vi "ValidateConfig.vi"(8 "error in (no error)":errorcluster, 11 "Channel in":refnum<class "Channel.lvclass">) -> (0 "error out":errorcluster, 2 "valid?":bool, 3 "Channel out":refnum<class "Channel.lvclass">)   [LabVIEW 2018, in "Channel.lvclass"]
uses:
  Channel.lvclass
  Channel.lvclass/Channel.ctl
  Interface/Interface.lvclass/Interface.ctl
  Interface/Interface.lvclass
panel:
  # "T=valid\nF=error"
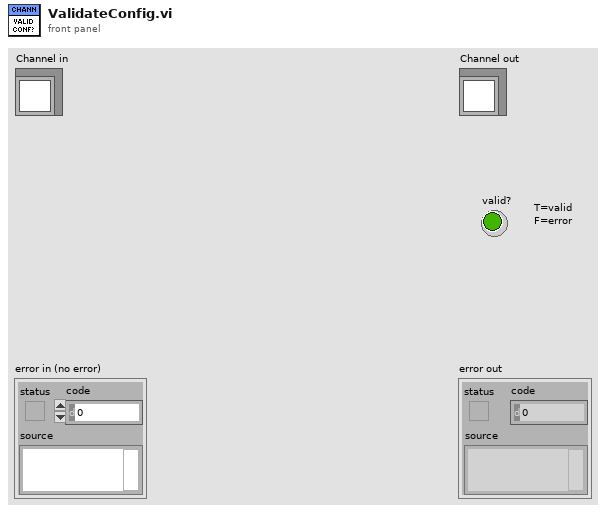
[diagram p1: front panel]
types:
  T1 = cluster{"ACQUISITION_MODE":u8, "TRIGGER_MODE":u8, "READ_MODE":u8, "PREAMP":u8, "READOUT_RATE":u8, "VERTICAL_SHIFT_SPEED":u8, "EM_MODE":u8, "EM_GAIN":u16, "SHUTTER_MODE":u8, "SHUTTER_TTL":u8, "SHUTTER_OPENING_TIME":u16, "SHUTTER_CLOSING_TIME":u16, "VBIN":u16, "HBIN":u16, "INITIAL_LINE":u16, "INITIAL_COLUMN":u16, "FINAL_LINE":u16, "FINAL_COLUMN":u16, "FRAME_TRANSFER":bool, "VERTICAL_CLOCK_VOLTAGE":u8, "AD_CHANNEL":u32}
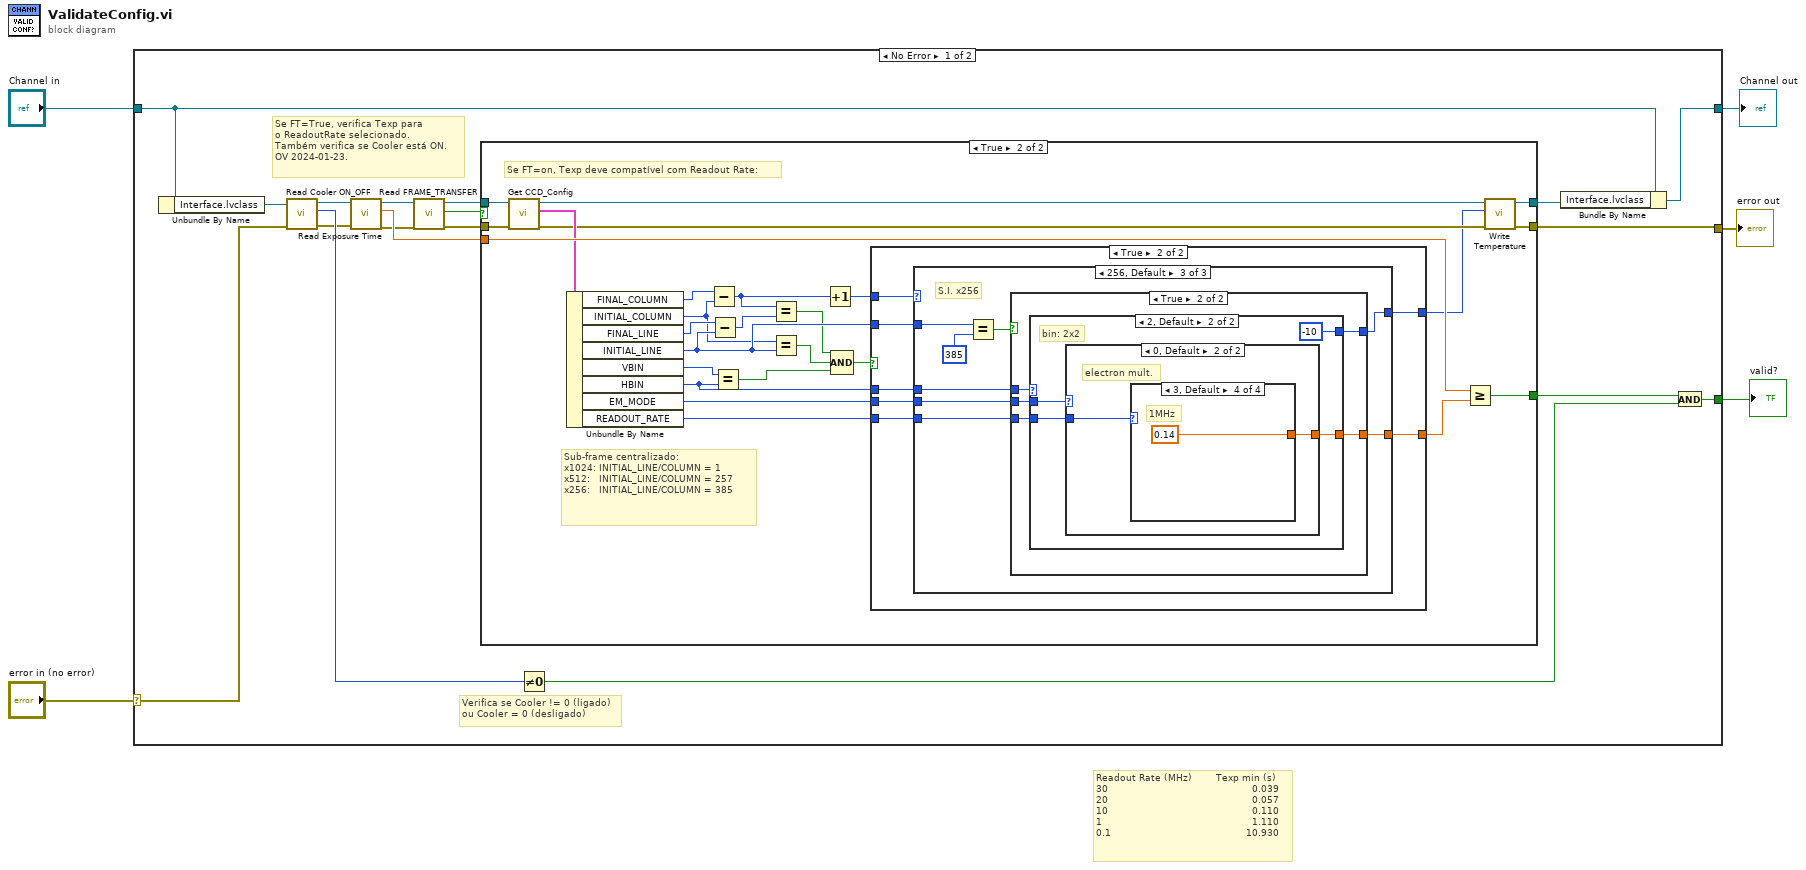
[diagram p0: block diagram]
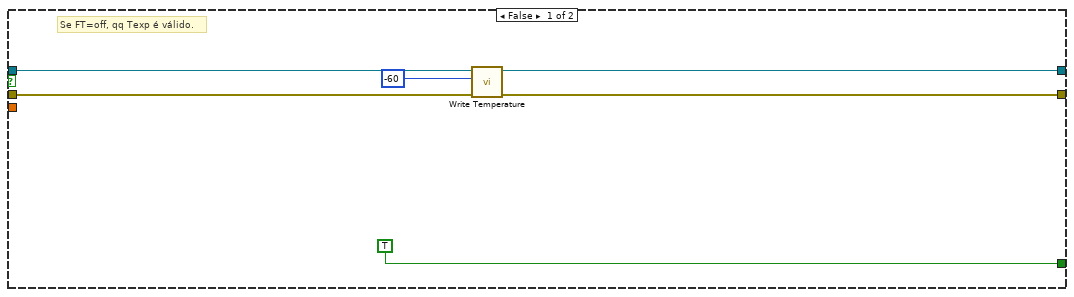
[diagram p2: hidden frame]
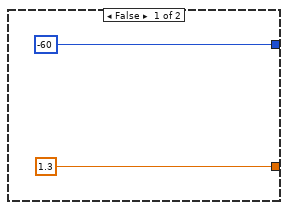
[diagram p3: hidden frame]
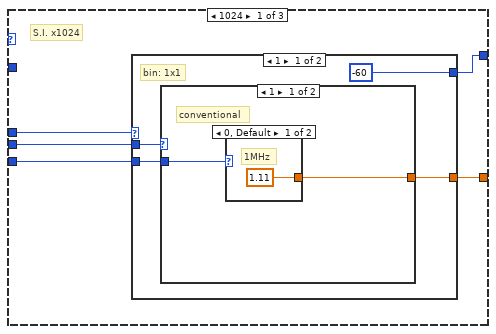
[diagram p4: hidden frame]
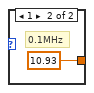
[diagram p5: hidden frame]
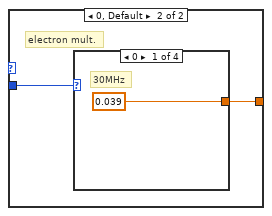
[diagram p6: hidden frame]
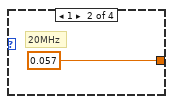
[diagram p7: hidden frame]
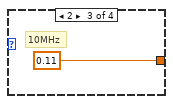
[diagram p8: hidden frame]
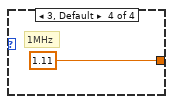
[diagram p9: hidden frame]
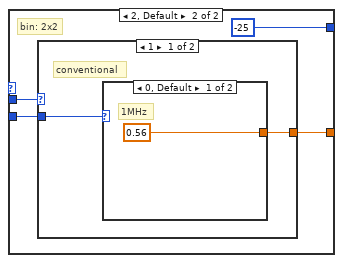
[diagram p10: hidden frame]
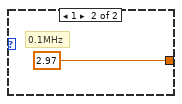
[diagram p11: hidden frame]
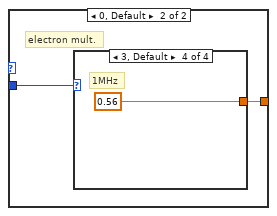
[diagram p12: hidden frame]
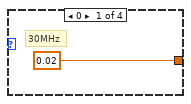
[diagram p13: hidden frame]
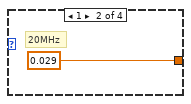
[diagram p14: hidden frame]
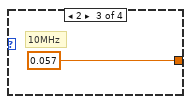
[diagram p15: hidden frame]
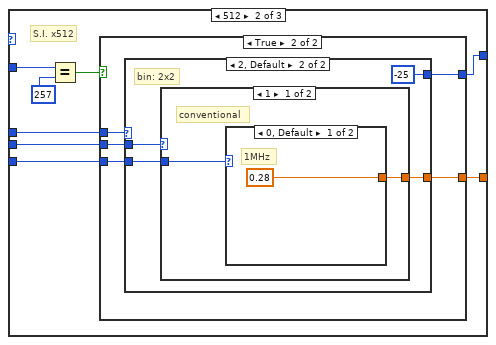
[diagram p16: hidden frame]
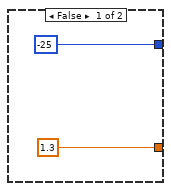
[diagram p17: hidden frame]
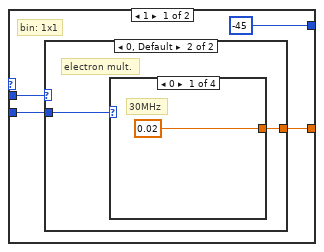
[diagram p18: hidden frame]
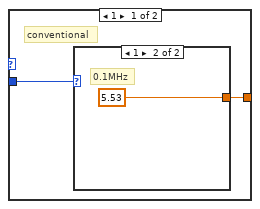
[diagram p19: hidden frame]
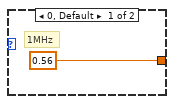
[diagram p20: hidden frame]
diagram:
  # "Readout Rate (MHz)        Texp min (s)\n30                                                0.039\n20                                                0.057  \n10                                                0.110\n1                                                  1.110\n0.1                                             10.930"
  n1 = case shown="No Error" "error in (no error)" {
    selector: "error in (no error)" -> [w17 w186]
    tunnel: [w9 w186] -> w4
    tunnel: [w7 w185] -> w2
    tunnel: "Channel in" -> [w8 w185]
    tunnel: [w14 FALSE] -> w1
    frame No Error {
      # "Verifica se Cooler != 0 (ligado)\nou Cooler = 0 (desligado)"
      # "Se FT=True, verifica Texp para \no ReadoutRate selecionado.\nTambém verifica se Cooler está ON.\nOV 2024-01-23."
      n2 = Unbundle By Name(w8) -> ("Interface.lvclass"=w20:refnum<class "Interface.lvclass">)
      n3 = call-dynamic "Read Cooler ON_OFF.vi"("error in (no error)"=w17, "Interface in"=w20) -> ("error out"=w16:errorcluster, "Cooler ON/OFF"=w18:i16, "Interface out"=w19:refnum<class "Interface.lvclass">)  [unwired: 7 in]
      n4 = call "Read Exposure Time.vi"("error in (no error)"=w16, "Interface in"=w19) -> ("error out"=w15:errorcluster, "Exposure Time"=w21:dbl, "Interface out"=w23:refnum<class "Interface.lvclass">)  [unwired: 7 in]
      n5 = call-dynamic "Read FRAME_TRANSFER.vi"("error in (no error)"=w15, "Interface in"=w23) -> ("error out"=w10:errorcluster, "FRAME_TRANSFER"=w22:bool, "Interface out"=w11:refnum<class "Interface.lvclass">)  [unwired: 7 in]
      n6 = case shown="True" w22 {
        tunnel: w21 -> [_ w55]
        tunnel: [TRUE w53] -> w13
        tunnel: w11 -> [w27 w51]
        tunnel: w10 -> [w28 w50]
        tunnel: [w25 w37] -> w9
        tunnel: [w26 w34] -> w6
        frame False {
          # "Se FT=off, qq Texp é válido."
          n7 = call-dynamic "Write Temperature.vi"("error in (no error)"=w28, "Temperature"=i8 -60, "Interface in"=w27) -> ("error out"=w25:errorcluster, "Interface out"=w26:refnum<class "Interface.lvclass">)  [unwired: 7 in]
        }
        frame True {
          # "Sub-frame centralizado:\nx1024: INITIAL_LINE/COLUMN = 1\nx512:   INITIAL_LINE/COLUMN = 257\nx256:   INITIAL_LINE/COLUMN = 385"
          # "Se FT=on, Texp deve compatível com Readout Rate:"
          n8 = call-dynamic "Get CCD_Config.vi"("error in (no error)"=w50, "Interface in"=w51) -> ("error out"=w38:errorcluster, "output cluster"=w52:T1, "Interface out"=w35:refnum<class "Interface.lvclass">)  [unwired: 7 in]
          n9 = Unbundle By Name(w52) -> ("FINAL_COLUMN"=w47:u16, "INITIAL_COLUMN"=w32:u16, "FINAL_LINE"=w46:u16, "INITIAL_LINE"=w33:u16, "VBIN"=w44:u16, "HBIN"=w40:u16, "EM_MODE"=w49:u8, "READOUT_RATE"=w48:u8)
          n10 = Subtract(x=w47, y=w32) -> (x-y=w41:u16)
          n11 = Subtract(x=w46, y=w33) -> (x-y=w45:u16)
          n12 = Equal?(x=w44, y=w40) -> (x = y?=w42:bool)
          n13 = Equal?(x=w41, y=w45) -> (x = y?=w31:bool)
          n14 = Equal?(x=w32, y=w33) -> (x = y?=w30:bool)
          n15 = Increment(x=w41) -> (x+1=w39:u16)
          n16 = Compound Arithmetic op=AND(w31, w30, w42) -> (w43:bool)
          n17 = case shown="True" w43 {
            tunnel: [1.3 ("y") w64] -> w54
            tunnel: w49 -> [_ w63]
            tunnel: w48 -> [_ w62]
            tunnel: w39 -> [_ w61]
            tunnel: w40 -> [_ w60]
            tunnel: [i8 -60 ("y") w59] -> w36
            tunnel: w33 -> [_ w58]
            frame False {
            }
            frame True {
              n18 = case shown="256, Default" w61 {
                tunnel: [w69 w105 w148] -> w64
                tunnel: w63 -> [w68 w104 w147]
                tunnel: w62 -> [w67 w103 w146]
                tunnel: w60 -> [w66 w102 w145]
                tunnel: [w65 w101 w144] -> w59
                tunnel: w58 -> [_ w100 w142]
                frame 1024 {
                  # "S.I. x1024"
                  n19 = case shown="1" w66 {
                    tunnel: [w73 w87] -> w69
                    tunnel: w68 -> [w72 w86]
                    tunnel: w67 -> [w71 w85]
                    tunnel: [i8 -60 ("y") i8 -25 ("y")] -> w65
                    frame 1 {
                      # "bin: 1x1"
                      n20 = case shown="1" w72 {
                        tunnel: [w75 w79] -> w73
                        tunnel: w71 -> [w74 w78]
                        frame 1 {
                          # "conventional"
                          n21 = case shown="0, Default" w74 {
                            tunnel: [1.11 ("y") 10.93 ("y")] -> w75
                            frame 0, Default {
                              # "1MHz"
                            }
                            frame 1 {
                              # "0.1MHz"
                            }
                          }
                        }
                        frame 0, Default {
                          # "electron mult."
                          n22 = case shown="0" w78 {
                            tunnel: [0.039 ("y") 0.057 ("y") 0.11 ("y") 1.11 ("y")] -> w79
                            frame 0 {
                              # "30MHz"
                            }
                            frame 1 {
                              # "20MHz"
                            }
                            frame 2 {
                              # "10MHz"
                            }
                            frame 3, Default {
                              # "1MHz"
                            }
                          }
                        }
                      }
                    }
                    frame 2, Default {
                      # "bin: 2x2"
                      n23 = case shown="1" w86 {
                        tunnel: [w89 w93] -> w87
                        tunnel: w85 -> [w88 w92]
                        frame 1 {
                          # "conventional"
                          n24 = case shown="0, Default" w88 {
                            tunnel: [0.56 ("y") 2.97 ("y")] -> w89
                            frame 0, Default {
                              # "1MHz"
                            }
                            frame 1 {
                              # "0.1MHz"
                            }
                          }
                        }
                        frame 0, Default {
                          # "electron mult."
                          n25 = case shown="3, Default" w92 {
                            tunnel: [0.02 ("y") 0.029 ("y") 0.057 ("y") 0.56 ("y")] -> w93
                            frame 0 {
                              # "30MHz"
                            }
                            frame 1 {
                              # "20MHz"
                            }
                            frame 2 {
                              # "10MHz"
                            }
                            frame 3, Default {
                              # "1MHz"
                            }
                          }
                        }
                      }
                    }
                  }
                }
                frame 512 {
                  # "S.I. x512"
                  n26 = Equal?(x=w100, y=u16 257) -> (x = y?=w98:bool)
                  n27 = case shown="True" w98 {
                    tunnel: [1.3 ("y") w112] -> w105
                    tunnel: w104 -> [_ w111]
                    tunnel: w103 -> [_ w110]
                    tunnel: w102 -> [_ w109]
                    tunnel: [i8 -25 ("y") w108] -> w101
                    frame False {
                    }
                    frame True {
                      n28 = case shown="2, Default" w109 {
                        tunnel: [w116 w130] -> w112
                        tunnel: w111 -> [w115 w129]
                        tunnel: w110 -> [w114 w128]
                        tunnel: [i8 -45 ("y") i8 -25 ("y")] -> w108
                        frame 1 {
                          # "bin: 1x1"
                          n29 = case shown="0, Default" w115 {
                            tunnel: [w118 w122] -> w116
                            tunnel: w114 -> [w117 w121]
                            frame 1 {
                              # "conventional"
                              n30 = case shown="1" w117 {
                                tunnel: [0.56 ("y") 5.53 ("y")] -> w118
                                frame 0, Default {
                                # "1MHz"
                                }
                                frame 1 {
                                # "0.1MHz"
                                }
                              }
                            }
                            frame 0, Default {
                              # "electron mult."
                              n31 = case shown="0" w121 {
                                tunnel: [0.02 ("y") 0.029 ("y") 0.057 ("y") 0.56 ("y")] -> w122
                                frame 0 {
                                # "30MHz"
                                }
                                frame 1 {
                                # "20MHz"
                                }
                                frame 2 {
                                # "10MHz"
                                }
                                frame 3, Default {
                                # "1MHz"
                                }
                              }
                            }
                          }
                        }
                        frame 2, Default {
                          # "bin: 2x2"
                          n32 = case shown="1" w129 {
                            tunnel: [w132 w136] -> w130
                            tunnel: w128 -> [w131 w135]
                            frame 1 {
                              # "conventional"
                              n33 = case shown="0, Default" w131 {
                                tunnel: [0.28 ("y") 2.14 ("y")] -> w132
                                frame 0, Default {
                                # "1MHz"
                                }
                                frame 1 {
                                # "0.1MHz"
                                }
                              }
                            }
                            frame 0, Default {
                              # "electron mult."
                              n34 = case shown="3, Default" w135 {
                                tunnel: [0.011 ("y") 0.015 ("y") 0.029 ("y") 0.28 ("y")] -> w136
                                frame 0 {
                                # "30MHz"
                                }
                                frame 1 {
                                # "20MHz"
                                }
                                frame 2 {
                                # "10MHz"
                                }
                                frame 3, Default {
                                # "1MHz"
                                }
                              }
                            }
                          }
                        }
                      }
                    }
                  }
                }
                frame 256, Default {
                  # "S.I. x256"
                  n35 = Equal?(x=w142, y=u16 385) -> (x = y?=w141:bool)
                  n36 = case shown="True" w141 {
                    tunnel: [1.3 ("y") w155] -> w148
                    tunnel: w147 -> [_ w154]
                    tunnel: w146 -> [_ w153]
                    tunnel: w145 -> [_ w152]
                    tunnel: [i8 -10 ("y") w151] -> w144
                    frame False {
                    }
                    frame True {
                      n37 = case shown="2, Default" w152 {
                        tunnel: [w159 w173] -> w155
                        tunnel: w154 -> [w158 w172]
                        tunnel: w153 -> [w157 w171]
                        tunnel: [i8 -33 ("y") i8 -10 ("y")] -> w151
                        frame 1 {
                          # "bin: 1x1"
                          n38 = case shown="0, Default" w158 {
                            tunnel: [w161 w165] -> w159
                            tunnel: w157 -> [w160 w164]
                            frame 1 {
                              # "conventional"
                              n39 = case shown="0, Default" w160 {
                                tunnel: [0.28 ("y") 2.79 ("y")] -> w161
                                frame 0, Default {
                                # "1MHz"
                                }
                                frame 1 {
                                # "0.1MHz"
                                }
                              }
                            }
                            frame 0, Default {
                              # "electron mult."
                              n40 = case shown="1" w164 {
                                tunnel: [0.011 ("y") 0.015 ("y") 0.029 ("y") 0.28 ("y")] -> w165
                                frame 0 {
                                # "30MHz"
                                }
                                frame 1 {
                                # "20MHz"
                                }
                                frame 2 {
                                # "10MHz"
                                }
                                frame 3, Default {
                                # "1MHz"
                                }
                              }
                            }
                          }
                        }
                        frame 2, Default {
                          # "bin: 2x2"
                          n41 = case shown="0, Default" w172 {
                            tunnel: [w175 w179] -> w173
                            tunnel: w171 -> [w174 w178]
                            frame 1 {
                              # "conventional"
                              n42 = case shown="0, Default" w174 {
                                tunnel: [0.14 ("y") 1.24 ("y")] -> w175
                                frame 0, Default {
                                # "1MHz"
                                }
                                frame 1 {
                                # "0.1MHz"
                                }
                              }
                            }
                            frame 0, Default {
                              # "electron mult."
                              n43 = case shown="3, Default" w178 {
                                tunnel: [0.0059 ("y") 0.0083 ("y") 0.015 ("y") 0.14 ("y")] -> w179
                                frame 0 {
                                # "30MHz"
                                }
                                frame 1 {
                                # "20MHz"
                                }
                                frame 2 {
                                # "10MHz"
                                }
                                frame 3, Default {
                                # "1MHz"
                                }
                              }
                            }
                          }
                        }
                      }
                    }
                  }
                }
              }
            }
          }
          n44 = Greater Or Equal?(x=w55, y=w54) -> (x >= y?=w53:bool)
          n45 = call-dynamic "Write Temperature.vi"("error in (no error)"=w38, "Temperature"=w36, "Interface in"=w35) -> ("error out"=w37:errorcluster, "Interface out"=w34:refnum<class "Interface.lvclass">)  [unwired: 7 in]
        }
      }
      n46 = Not Equal To 0?(x=w18) -> (x != 0?=w12:bool)
      n47 = Bundle By Name(cluster=w8, "Interface.lvclass"=w6) -> (w7:refnum<class "Channel.lvclass">)
      n48 = And(x=w13, y=w12) -> (x .and. y?=w14:bool)
    }
    frame Error {
    }
  }
  "error out" <- w4
  "Channel out" <- w2
  "valid?" <- w1
